vi "Select Shape.vi"(11 "Numeric":i32) -> (3 "Shape":string[][](array[string]))   [LabVIEW 2021]
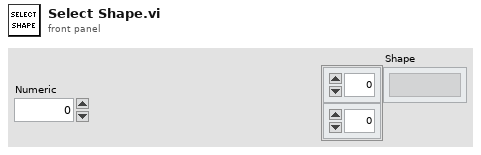
[diagram p1: front panel]
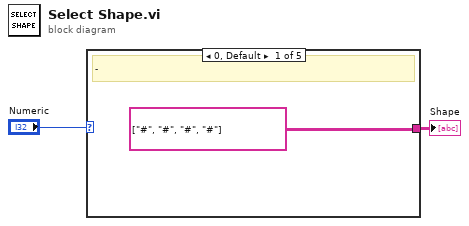
[diagram p0: block diagram]
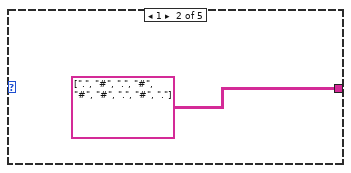
[diagram p2: hidden frame]
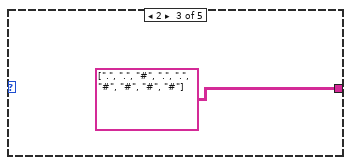
[diagram p3: hidden frame]
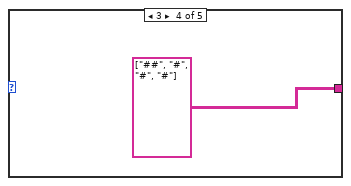
[diagram p4: hidden frame]
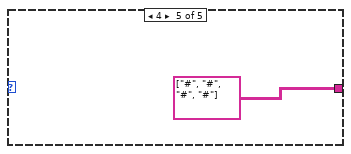
[diagram p5: hidden frame]
diagram:
  n1 = case shown="0, Default" "Numeric" {
    tunnel: [string[][] [["#", "#", "#", "#"]] string[][] [[".", "#", "."], ["#", "#", "#"], [".", "#", "."]] string[][] [[".", ".", "#"], [".", ".", "#"], ["#", "#", "#"]] string[][] [["##"], ["#"], ["#"], ["#"]] string[][] [["#", "#"], ["#", "#"]]] -> w1
    frame 0, Default {
      # "-"
    }
    frame 1 {
    }
    frame 2 {
    }
    frame 3 {
    }
    frame 4 {
    }
  }
  "Shape" <- w1
